vi "Manage Collision.vi"(11 "Ball-Ball in":refnum<class "Ball-Ball.lvclass">) -> (1 "Remove GB Components out":refnum<class "Game Board Component.lvclass">[](array[class]), 2 "GB Components out":refnum<class "Game Board Component.lvclass">[](array[class]))   [LabVIEW 2024, in "Ball-Ball.lvclass"]
doc: "MIT Licence\nCopyright (c) 2024 David Grollier"
uses:
  Ball-Ball.lvclass
  Game Componants/Game Board Component/Game Board Component.lvclass
  Game Componants/Game Board Component/Movable/Movable.lvclass
  Collision.lvclass/Collision.ctl
  Game Componants/Game Board Component/Movable/Movable.lvclass/Movable.ctl
  Game Componants/Game Componants.lvclass/Game Componants.ctl
  Game Componants/Game Board/Game Board.lvclass
  Game Componants/Game Componants.lvclass
  Collision.lvclass
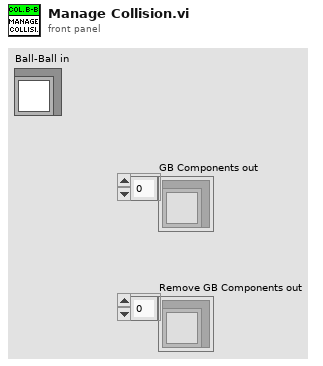
[diagram p1: front panel]
types:
  T1 = typedef "Velocity.ctl" = cluster{"Vx":dbl, "Vy":dbl}
  T2 = typedef "Coordinates.ctl" = cluster{"x":dbl, "y":dbl}
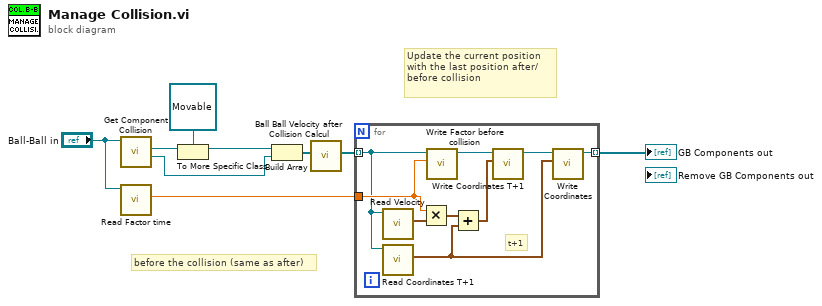
[diagram p0: block diagram]
diagram:
  # "before the collision (same as after)"
  # "Update the current position with the last position after/before collision"
  n1 = call "Get Component Collision.vi"("Collision in"="Ball-Ball in") -> ("Movable out"=w6:refnum<class "Movable.lvclass">, "GB Component out"=w7:refnum<class "Game Board Component.lvclass">)  [unwired: 9 in]
  n2 = call "Read Factor time.vi"("Collision in"="Ball-Ball in") -> ("Factor time"=w1:dbl)  [unwired: 10 in]
  n3 = To More Specific Class(target class=refnum<class "Movable.lvclass"> refnum ("specific class reference"), reference=w7) -> (specific class reference=w5:refnum<class "Movable.lvclass">)  [unwired: 1 in, 1 out]
  n4 = Build Array(w5, w6) -> (w4:refnum<class "Movable.lvclass">[])
  n5 = call "Ball Ball Velocity after Collision Calcul.vi"("Movables in"=w4) -> ("Movables out"=w9:refnum<class "Movable.lvclass">[])  [unwired: 10 in]
  n6 = for {
    tunnel: w9 -> [w12] mode=indexing
    tunnel: [w17] -> w3 mode=indexing
    tunnel: w1 -> [w13]
    # "t+1"
    n7 = call-dynamic "Read Velocity.vi"("Movable in"=w12) -> ("Velocity"=w16:T1)  [unwired: 10 in]
    n8 = call "Read Coordinates T+1.vi"("Movable in"=w12) -> ("Coordinates"=w15:T2)  [unwired: 10 in]
    n9 = Multiply(x=w13, y=w16) -> (x*y=w18:T1)
    n10 = call "Write Factor before collision.vi"("Factor before collision"=w13, "Movable in"=w12) -> ("Movable out"=w11:refnum<class "Movable.lvclass">)  [unwired: 9 in]
    n11 = Add(x=w18, y=w15) -> (x+y=w14:T1)
    n12 = call "Write Coordinates T+1.vi"("Coordinates"=w14, "Movable in"=w11) -> ("Movable out"=w10:refnum<class "Movable.lvclass">)  [unwired: 9 in]
    n13 = call "Write Coordinates.vi"("Coordinates"=w15, "Game Componants in"=w10) -> ("Game Componants out"=w17:refnum<class "Movable.lvclass">)  [unwired: 9 in]
  }
  "GB Components out" <- w3
